vi "Encoder_PanelSim_Global.vi"(0 "menu":T4=enum."set reset", 5 "EncoderIndex":T3, 7 "Value Set":bool, 9 "Numeric Value":dbl format="%#.4f", 11 "error in (no error)":errorcluster, 12 "String Value":string) -> (10 "Encoder new":T1={"type"="Encoder", "device"="", "name"="", "data"={"<init"=FALSE, ">count"=0.0, ">period"=0.0, "<samples_to_avg"=0, "<offset"=0.0, "<channel_a"=0, "<channel_b"=0}}, 15 "error out":errorcluster)   [LabVIEW 2019]
doc: "This is used to set and get the last motor output values. This is needed for simulation, since we cannot read these values from the hardware.\n\nThis software is licensed. Open the labview\\readme\\WPI Robotics Library Open Source License.txt file for more information."
uses:
  Encoder data protoo.ctl
  Encoder proto.ctl
  Encoder Update Ops.ctl
  <vilib>/Rock Robotics/SystemInterfaces/Encoder/FPGA_EncoderIdx.ctl
panel:
  out "All Values":T1[](array[typedef])
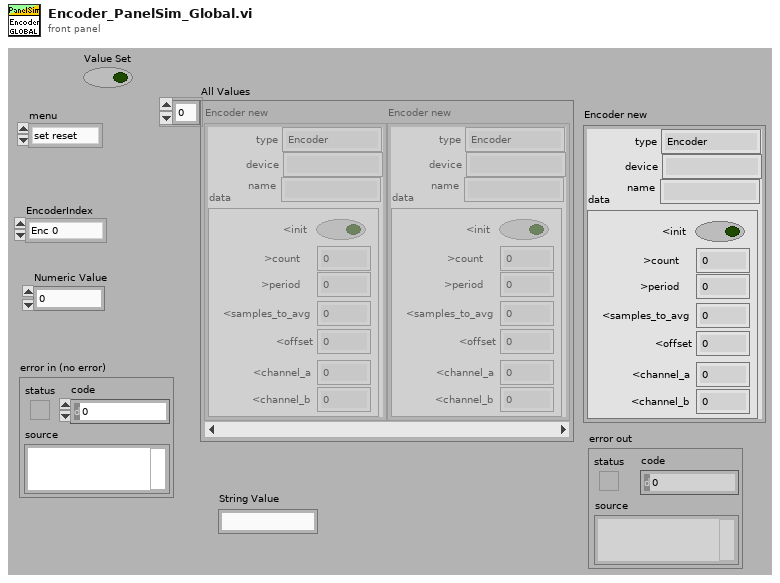
[diagram p1: front panel]
types:
  T1 = typedef "Encoder proto.ctl" = cluster{"type":string, "device":string, "name":string, "data":T2}
  T2 = typedef "Encoder data protoo.ctl" = cluster{"<init":bool, ">count":dbl, ">period":dbl, "<samples_to_avg":i32, "<offset":dbl, "<channel_a":i32, "<channel_b":i32}
  T3 = typedef "FPGA_EncoderIdx.ctl" = enum8{"Enc 0", "Enc 1", "Enc 2", "Enc 3", "Enc 4", "Enc 5", "Enc 6", "Enc 7", "Invalid"}
  T4 = typedef "Encoder Update Ops.ctl" = enum16{"set init", "set count", "set period", "set reset", "set samples_to_avg", "get", "delete", "JSON update", "set name", "transmit initial", "reset", "set channel_a", "set channel_b"}
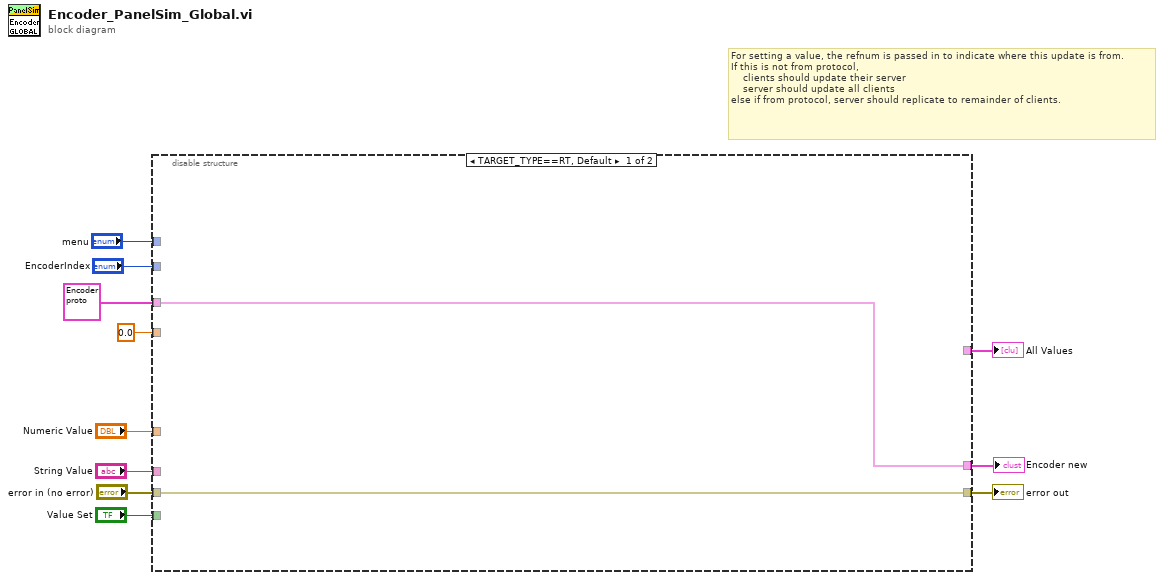
[diagram p0: block diagram]
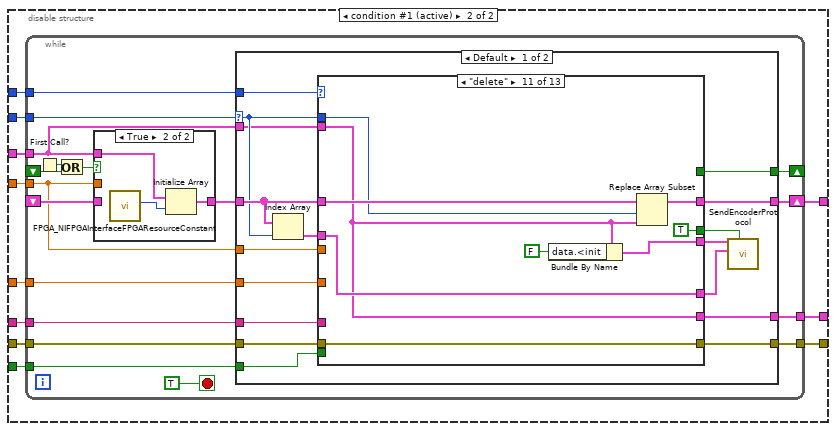
[diagram p2: hidden frame]
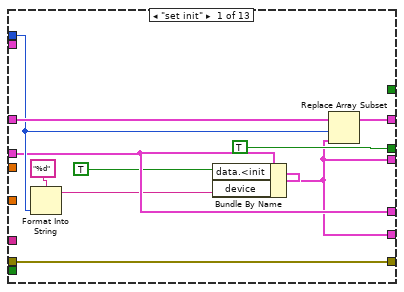
[diagram p3: hidden frame]
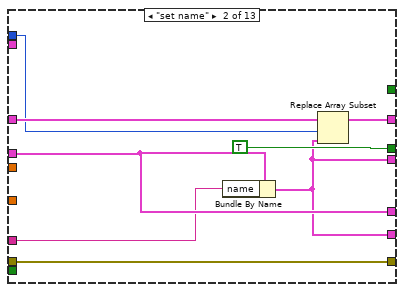
[diagram p4: hidden frame]
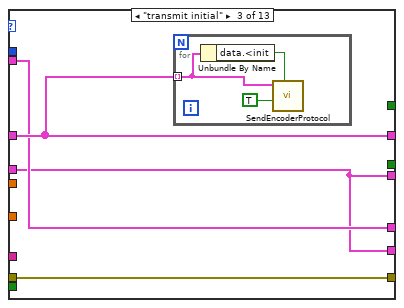
[diagram p5: hidden frame]
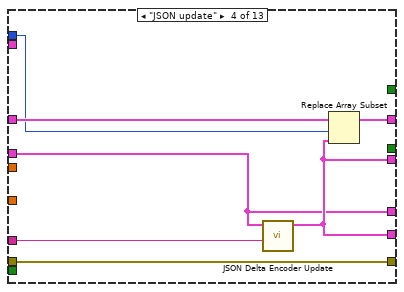
[diagram p6: hidden frame]
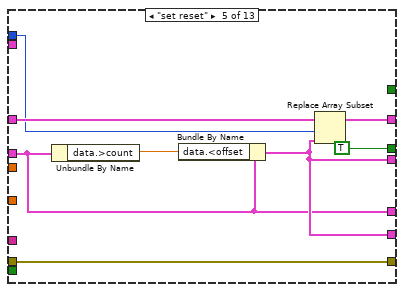
[diagram p7: hidden frame]
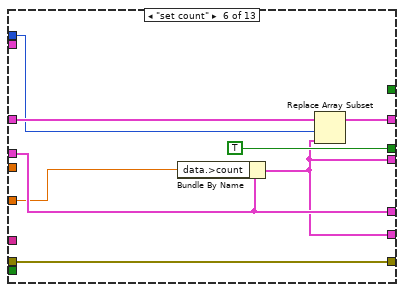
[diagram p8: hidden frame]
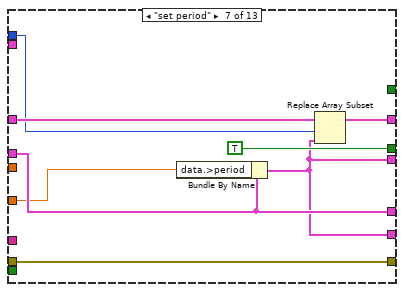
[diagram p9: hidden frame]
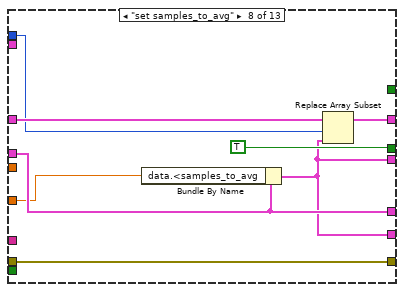
[diagram p10: hidden frame]
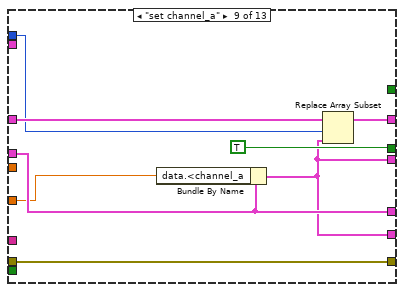
[diagram p11: hidden frame]
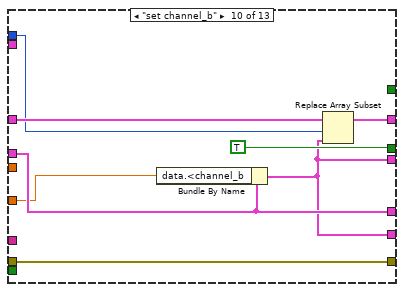
[diagram p12: hidden frame]
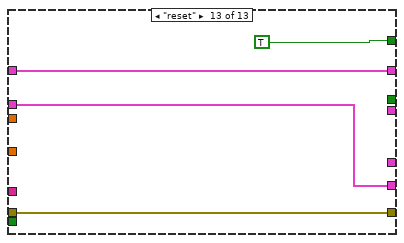
[diagram p14: hidden frame]
diagram:
  # "For setting a value, the refnum is passed in to indicate where this update is from.\nIf this is not from protocol,\n    clients should update their server\n    server should update all clients\nelse if from protocol, server should replicate to remainder of clients."
  n1 = disable-structure shown="TARGET_TYPE==RT, Default" {
    disable-tunnel: "menu" -> [_ w24]
    disable-tunnel: [w13 w23] -> w10
    disable-tunnel: "error in (no error)" -> [w13 w22]
    disable-tunnel: [_ w21] -> w8
    disable-tunnel: 0.0 ("Output") -> [_ w20]
    disable-tunnel: "EncoderIndex" -> [_ w19]
    disable-tunnel: [w12 w18] -> w5
    disable-tunnel: T1 {"type"="Encoder", "device"="", "name"="", "data"={"<init"=FALSE, ">count"=0.0, ">period"=0.0, "<samples_to_avg"=0, "<offset"=0.0, "<channel_a"=0, "<channel_b"=0}} ("Encoder new") -> [w12 w17]
    disable-tunnel: "String Value" -> [_ w16]
    disable-tunnel: "Numeric Value" -> [_ w15]
    disable-tunnel: "Value Set" -> [_ w14]
    frame condition #0 {
    }
    frame condition #1 (active) {
      n2 = while {
        tunnel: w22 -> [w39]
        shift-right: [w42] -> w21
        shift-left: _ -> [w35]
        tunnel: [w41] -> w18
        tunnel: w24 -> [w40]
        tunnel: [w38] -> w23
        tunnel: w19 -> [w33]
        tunnel: w20 -> [w34]
        tunnel: w17 -> [w32]
        tunnel: w16 -> [w31]
        tunnel: w15 -> [w30]
        tunnel: w14 -> [w29]
        shift-right: [w25] -> _
        shift-left: _ -> [w26]
        stop <- TRUE stop-if-true
        n3 = First Call?() -> (First Call?: T/F=w28:bool)
        n4 = Or(x=w28, y=w26) -> (x .or. y?=w27:bool)
        n5 = case shown="True" w27 {
          tunnel: [w159 w162] -> w36
          tunnel: w35 -> [w159 _]
          tunnel: w34 -> [_ _]
          tunnel: w32 -> [_ w161]
          frame False {
          }
          frame True {
            n6 = call <vilib>:"FPGA_NIFPGAInterfaceFPGAResourceConstant.vi"() -> ("NumberOfEncoders"=w160:u32)  [unwired: 11 out]
            n7 = Initialize Array(w161, w160) -> (w162:T1[])
          }
        }
        n8 = case shown="Default" w33 {
          selector: w33 -> [w52 _]
          tunnel: [w59 w158] -> w42
          tunnel: [w58 w156] -> w41
          tunnel: w40 -> [w57 _]
          tunnel: w39 -> [w56 w157]
          tunnel: [w55 w157] -> w38
          tunnel: w36 -> [w54 w158]
          tunnel: w34 -> [w53 _]
          tunnel: w32 -> [w50 w156]
          tunnel: w31 -> [w49 _]
          tunnel: w30 -> [w48 _]
          tunnel: w29 -> [w44 _]
          tunnel: [w43 _] -> w25
          frame Default {
            n9 = Index Array(array=w54, index=w52) -> (element=w51:T1)
            n10 = case shown="\"delete\"" w57 {
              tunnel: [w69 w77 w80 w91 w99 w107 w115 w123 w131 w139 w147 w151 w155] -> w59
              tunnel: w54 -> [w67 w75 w80 w89 w97 w105 w113 w121 w129 w137 w148 w151 w155]
              tunnel: [w60 w71 w78 w87 w94 w101 w109 w117 w125 w133 w142 w149 w153] -> w58
              tunnel: [w68 w76 w81 w90 w98 w106 w114 w122 w130 w138 w146 w150 w154] -> w55
              tunnel: w56 -> [w68 w76 w81 w90 w98 w106 w114 w122 w130 w138 w146 w150 w154]
              tunnel: w52 -> [w64 w73 _ w88 w95 w103 w111 w119 w127 w135 w143 _ _]
              tunnel: w53 -> [_ _ _ _ _ _ _ _ _ _ _ _ _]
              tunnel: [w60 w71 w78 w87 w94 w101 w109 w117 w125 w133 w141 _ _] -> w46
              tunnel: [w63 w72 w79 w85 w93 w102 w110 w118 w126 w134 w144 _ _] -> w45
              tunnel: [TRUE TRUE _ _ TRUE TRUE TRUE TRUE TRUE TRUE TRUE _ _] -> w47
              tunnel: w51 -> [w63 w72 w78 w85 w93 w102 w110 w118 w126 w134 w144 w149 w153]
              tunnel: w50 -> [_ _ w79 _ _ _ _ _ _ _ w142 _ _]
              tunnel: w49 -> [_ w70 _ w86 _ _ _ _ _ _ _ _ _]
              tunnel: w48 -> [_ _ _ _ _ w100 w108 w116 w124 w132 _ _ _]
              tunnel: w44 -> [_ _ _ _ _ _ _ _ _ _ _ _ _]
              tunnel: [_ _ _ _ _ _ _ _ _ _ _ _ TRUE] -> w43
              frame "set init" {
                n11 = Format Into String(format string="%d", w64) -> (resulting string=w61:string)  [unwired: 2 in, 1 out]
                n12 = Bundle By Name(cluster=w63, "data.<init"=TRUE, "device"=w61) -> (w60:T1)
                n13 = Replace Array Subset(array=w67, new element=w60, index=w64) -> (w69:T1[])
              }
              frame "set name" {
                n14 = Bundle By Name(cluster=w72, "name"=w70) -> (w71:T1)
                n15 = Replace Array Subset(array=w75, new element=w71, index=w73) -> (w77:T1[])
              }
              frame "transmit initial" {
                n16 = for {
                  tunnel: w80 -> [w82] mode=indexing
                  n17 = Unbundle By Name(w82) -> ("data.<init"=w84:bool)
                  n18 = call "SendEncoderProtocol.vi"("Send"=w84, "Initialize"=TRUE, "Encoder new"=w82) -> ()  [unwired: 9 in]
                }
              }
              frame "JSON update" {
                n19 = call "JSON Delta Encoder Update.vi"("Delta JSON"=w86, "input"=w85) -> ("output"=w87:T1)  [unwired: 8 in, 1 out]
                n20 = Replace Array Subset(array=w89, new element=w87, index=w88) -> (w91:T1[])
              }
              frame "set reset" {
                n21 = Unbundle By Name(w93) -> ("data.>count"=w92:dbl)
                n22 = Bundle By Name(cluster=w93, "data.<offset"=w92) -> (w94:T1)
                n23 = Replace Array Subset(array=w97, new element=w94, index=w95) -> (w99:T1[])
              }
              frame "set count" {
                n24 = Bundle By Name(cluster=w102, "data.>count"=w100) -> (w101:T1)
                n25 = Replace Array Subset(array=w105, new element=w101, index=w103) -> (w107:T1[])
              }
              frame "set period" {
                n26 = Bundle By Name(cluster=w110, "data.>period"=w108) -> (w109:T1)
                n27 = Replace Array Subset(array=w113, new element=w109, index=w111) -> (w115:T1[])
              }
              frame "set samples_to_avg" {
                n28 = Bundle By Name(cluster=w118, "data.<samples_to_avg"=w116) -> (w117:T1)
                n29 = Replace Array Subset(array=w121, new element=w117, index=w119) -> (w123:T1[])
              }
              frame "set channel_a" {
                n30 = Bundle By Name(cluster=w126, "data.<channel_a"=w124) -> (w125:T1)
                n31 = Replace Array Subset(array=w129, new element=w125, index=w127) -> (w131:T1[])
              }
              frame "set channel_b" {
                n32 = Bundle By Name(cluster=w134, "data.<channel_b"=w132) -> (w133:T1)
                n33 = Replace Array Subset(array=w137, new element=w133, index=w135) -> (w139:T1[])
              }
              frame "delete" {
                n34 = Bundle By Name(cluster=w142, "data.<init"=FALSE) -> (w141:T1)
                n35 = Replace Array Subset(array=w148, new element=w142, index=w143) -> (w147:T1[])
              }
              frame "get" {
              }
              frame "reset" {
              }
            }
            n36 = call "SendEncoderProtocol.vi"("Send"=w47, "Encoder old"=w45, "Encoder new"=w46) -> ()  [unwired: 9 in]
          }
          frame "Invalid" {
            # "Do nothing if \nchannel is Invalid."
          }
        }
      }
    }
  }
  "error out" <- w10
  "All Values" <- w8
  "Encoder new" <- w5
